vi "Detect Saccades (Messy w Graph).vi"(8 "error in (no error)":errorcluster, 9 "Config":T1={"N Samples"=10, "Thresh Acc Min"=2000.0, "Thresh Acc Mult"=1.3, "Biphasic Condition"=1.5} {"Biphasic Condition" format="%#_13g"; "Thresh Acc Min" format="%#_13g"}, 10 "Sample Rate (Hz)":dbl=500.0, 11 "Velocity Data":dbl[](array[numeric])=[4.667303200298225, 4.909677731146953, 5.2109745814792365, 5.55763581565099, 5.920839247626144, 6.2599375275868905, 6.53696746567776, 6.72865184750785, 6.832732456031344, 6.865145184809078, 6.858206597001612, 6.855560991647909, 6.9019024854844275, 7.042027036538185, 7.301808557734746, 7.67879884433365, 8.162701363544402, 8.739894904566324, 9.381804070066359, 10.060971955287894, 10.76783422583134, 11.502246410072347, 12.262929879380705, 13.045081013541676, 13.853884817610783, 14.695951720056332, 15.571765573591499, 16.488535497561312, 17.454938324359695, 18.484011737786314, 19.593891983853432, 20.806854336741793, 22.151712241900537, 23.654011428085493, 25.337827690951034, 27.230327185694577, 29.362424125147363, 31.75316688648706, 34.39263748770516, 37.23987577100237, 40.20998271205074, 43.18048939513237, 46.018360137909205, 48.61044269433803, 50.91951950237008, 53.06311795006367, 55.36174711261601, 58.34239623139827, 62.72019604358697, 69.31912993124544, 78.92734080431808, 92.11979839547627, 109.07789039502565, 129.463835379339, 152.35306948148417, 176.24888250277527, 199.24480922686814, 219.27781203835607, 234.41475989201246, 243.14123432233515, 244.61162292671878, 238.79626072654116, 226.47186493405752, 209.08996299834854, 188.54095925571488, 166.85076670397655, 145.88590014607087, 127.10744294855878, 111.41329184954873, 99.10408789193212, 89.94838177953986, 83.32435573521803, 78.40945230557072, 74.36256040478978, 70.48301661914127, 66.30206830018594, 61.60225100109197, 56.40307274892831, 50.896616982148316, 45.35594505323262, 40.04915633283459, 35.188143251090374, 30.904438051178893, 27.239307747637383, 24.160247711926996, 21.591099822449937, 19.444244062457226, 17.63526417873216, 16.092631691774315, 14.772784905414664, 13.652421403949939, 12.714696659266576, 11.949486890601628, 11.345398431951562, 10.88883280531385, 10.5770353190049, 10.405836535787293, 10.356779466571126, 10.406311733622601, 10.524935218461192, 10.678830860111066, 10.826005759205444, 10.907035432214682, 10.871451934497463, 10.694375519365607, 10.368230576729, 9.920494644655006, 9.421715176905362, 8.966350342238707, 8.642097141771771, 8.514860672075699, 8.617942426550648, 8.924287001994747, 9.353183534744435, 9.799968965203188, 10.152498912607701, 10.316635671318952, 10.249410666570771, 9.96446844667745, 9.529806688600937, 9.047812081889603, 8.616326801793129, 8.303617903780026, 8.136163116655617, 8.097459448535563, 8.12521569051474, 8.127278177630815, 8.019623108839935, 7.7527652198374994, 7.3178418750367875, 6.743220089832729, 6.091225621655573, 5.4388335182966125, 4.852885740463117, 4.374362223112637, 4.008624562640419, 3.726319072887119, 3.471108403172712, 3.176519977519715, 2.78491418737247, 2.2594461410939903, 1.59493884099372, 0.8181822934693148, -0.026619214287534554, -0.8813264042654012, -1.6754180023234415, -2.342793907914615, -2.8391064532580135, -3.1473600057829927, -3.2704346606176187, -3.2194026522732617, -3.015049071127091, -2.6913407449721714, -2.288963866373292, -1.8552012819132093, -1.4426441696461185, -1.10637493868746, -0.9037185529715961, -0.8855105498645095, -1.0878872191121767, -1.5222387174285608, -2.1642000966113475, -2.948745621863602, -3.774741677175757, -4.521225848850843, -5.0658752955379045, -5.311170309597713, -5.208438257945705, -4.772561349308287, -4.075895907311848, -3.2362701273178054, -2.4080793800097897, -1.7480331896475167, -1.3703588224237055, -1.3200274321352738, -1.5735992621749766, -2.042730927283582, -2.5851998693665657, -3.037924337271747, -3.256090588254791, -3.148166973862299, -2.6984451055504195, -1.9731790520825205, -1.1065567390523348, -0.2681141821144437, 0.37409311669090695, 0.6891756583069366, 0.6155860122500014, 0.17941599326467195, -0.5082906845765738, -1.2803499480545852, -1.9480888478483216, -2.3401497209829145, -2.3440992169137296, -1.9281270895302551, -1.1459474421566647, -0.12830962259723222, 0.9363738210892123, 1.8357991288182767, 2.384599745817786, 2.4666064308939344, 2.054156463248786, 1.220863305309523, 0.12811068784634827, -1.018595010969218, -2.001752664406064, -2.6304649399676983, -2.7869433851410292, -2.4535594735302872, -1.7140485905140306, -0.7334883840388606, 0.27392426391968705, 1.094585023452499, 1.5568403033256075, 1.5611234362432445, 1.0986668385472989, 0.24684742597984943, -0.8452725331409354, -1.9880582489864462, -2.9877533974319324, -3.6879053692364785, -4.00617610589776, -3.9395155261628396, -3.5545628002925387, -2.964302429928681, -2.3045670045288436, -1.7128444883759233, -1.294689818423599, -1.105155718562152, -1.1485119963907628, -1.3895741513688282, -1.7715422803726764, -2.2274763350570232, -2.6932733895783443, -3.113940417779075, -3.45287905028652, -3.70267849231551, -3.8744215557206916, -3.9856590761507915, -4.052808173290114, -4.09332504597233, -4.127471814491399, -4.167454556957223, -4.213014549974331, -4.258926261854726, -4.300292567500452, -4.332119774166569, -4.355168465827725, -4.374979301903575, -4.394294193594332, -4.415209965022706, -4.441144186890184, -4.467481232862541, -4.483248995233593, -4.4855721436010825, -4.4746031408485205, -4.450689654707525, -4.422434151675683, -4.403223628429705, -4.405917482243676, -4.4399518225329295, -4.512143144357493, -4.622080929076186, -4.757550150950738, -4.8958998491602115, -5.008497957121103, -5.0656431974498695, -5.039159628319716, -4.911773985777418, -4.678249782158317]) -> (0 "error out":errorcluster, 3 "Saccades":T2[](array[typedef]))   [LabVIEW 2016]
uses:
  Type Definitions/Saccade Analyser Saccade Data.ctl
  <vilib>/Analysis/NI_AALPro.lvlib
  <vilib>/Analysis/NI_AAL_SigProc.lvlib
  <vilib>/ptbypt/NI_PtbyPt.lvlib
panel:
  out "XY Graph":cluster{"Ramp (s)":dbl[], "dX/dt":dbl[]}[](graph)
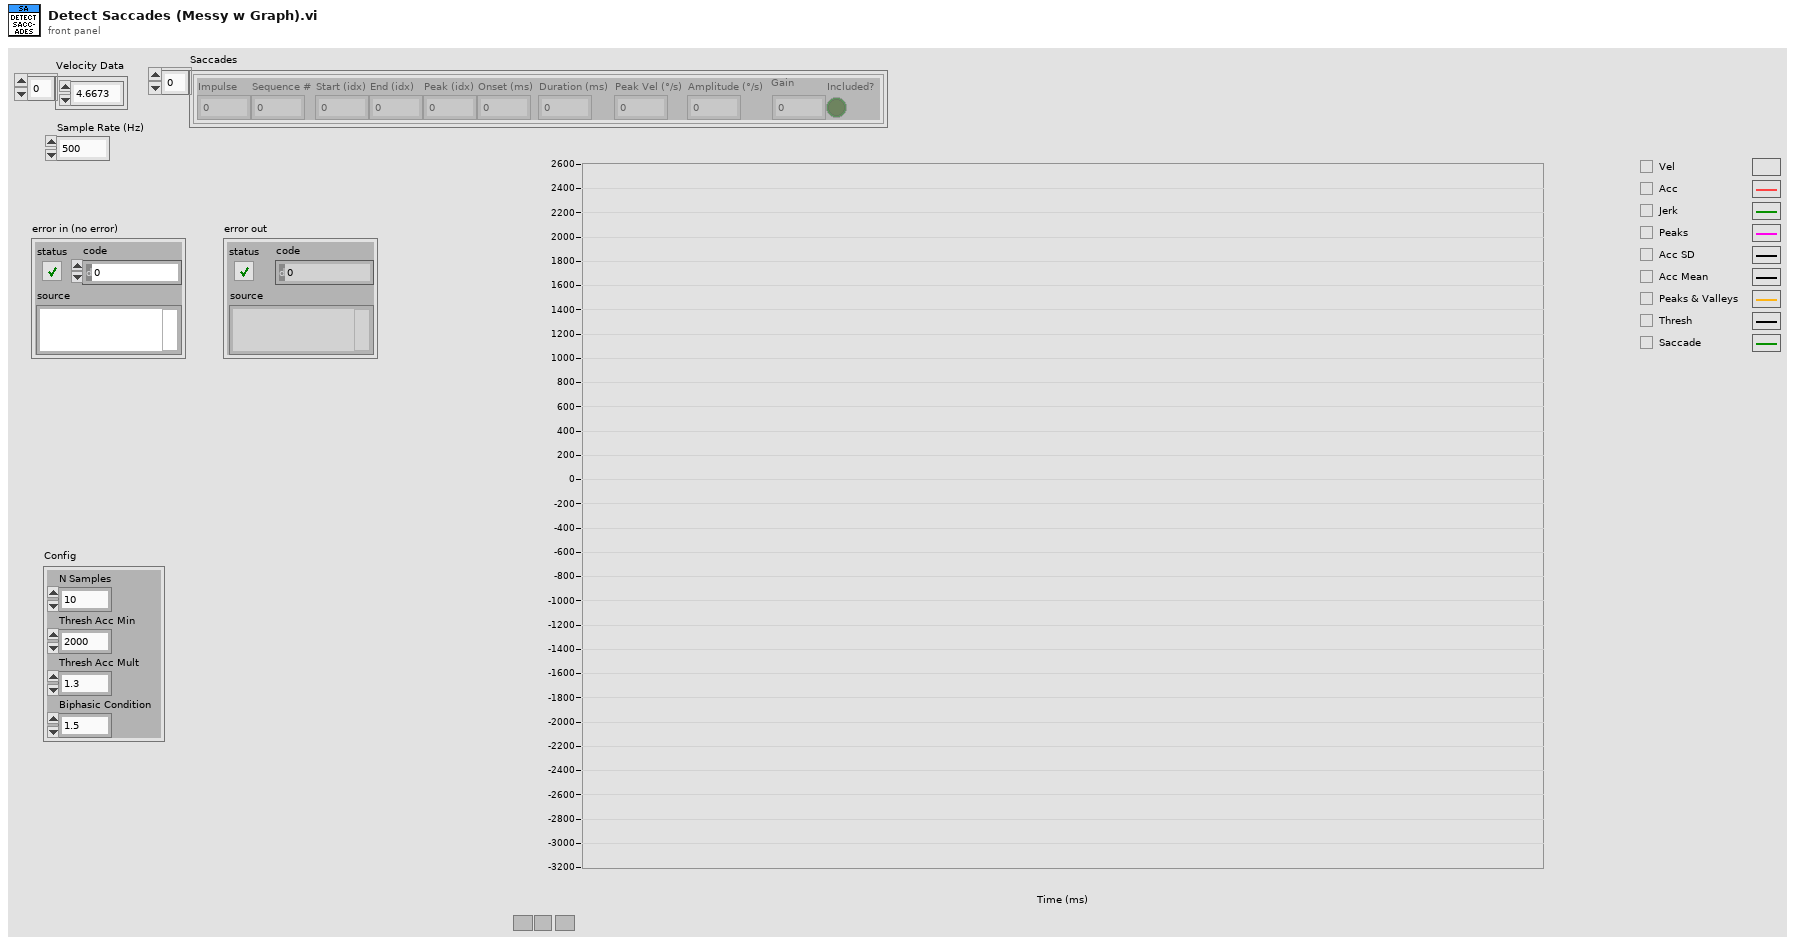
[diagram p1: front panel]
types:
  T1 = cluster{"N Samples":i32, "Thresh Acc Min":dbl, "Thresh Acc Mult":dbl, "Biphasic Condition":dbl}
  T2 = typedef "Saccade Analyser Saccade Data.ctl" = cluster{"Impulse":i32, "Sequence #":dbl, "Start (idx)":dbl, "End (idx)":dbl, "Peak (idx)":dbl, "Onset (ms)":dbl, "Duration (ms)":dbl, "Peak Vel (°/s)":dbl, "Amplitude (°/s)":dbl, "Gain":dbl, "Included?":bool}
  T3 = cluster{"Index":i32, "Peak?":bool, "Value":dbl}[]
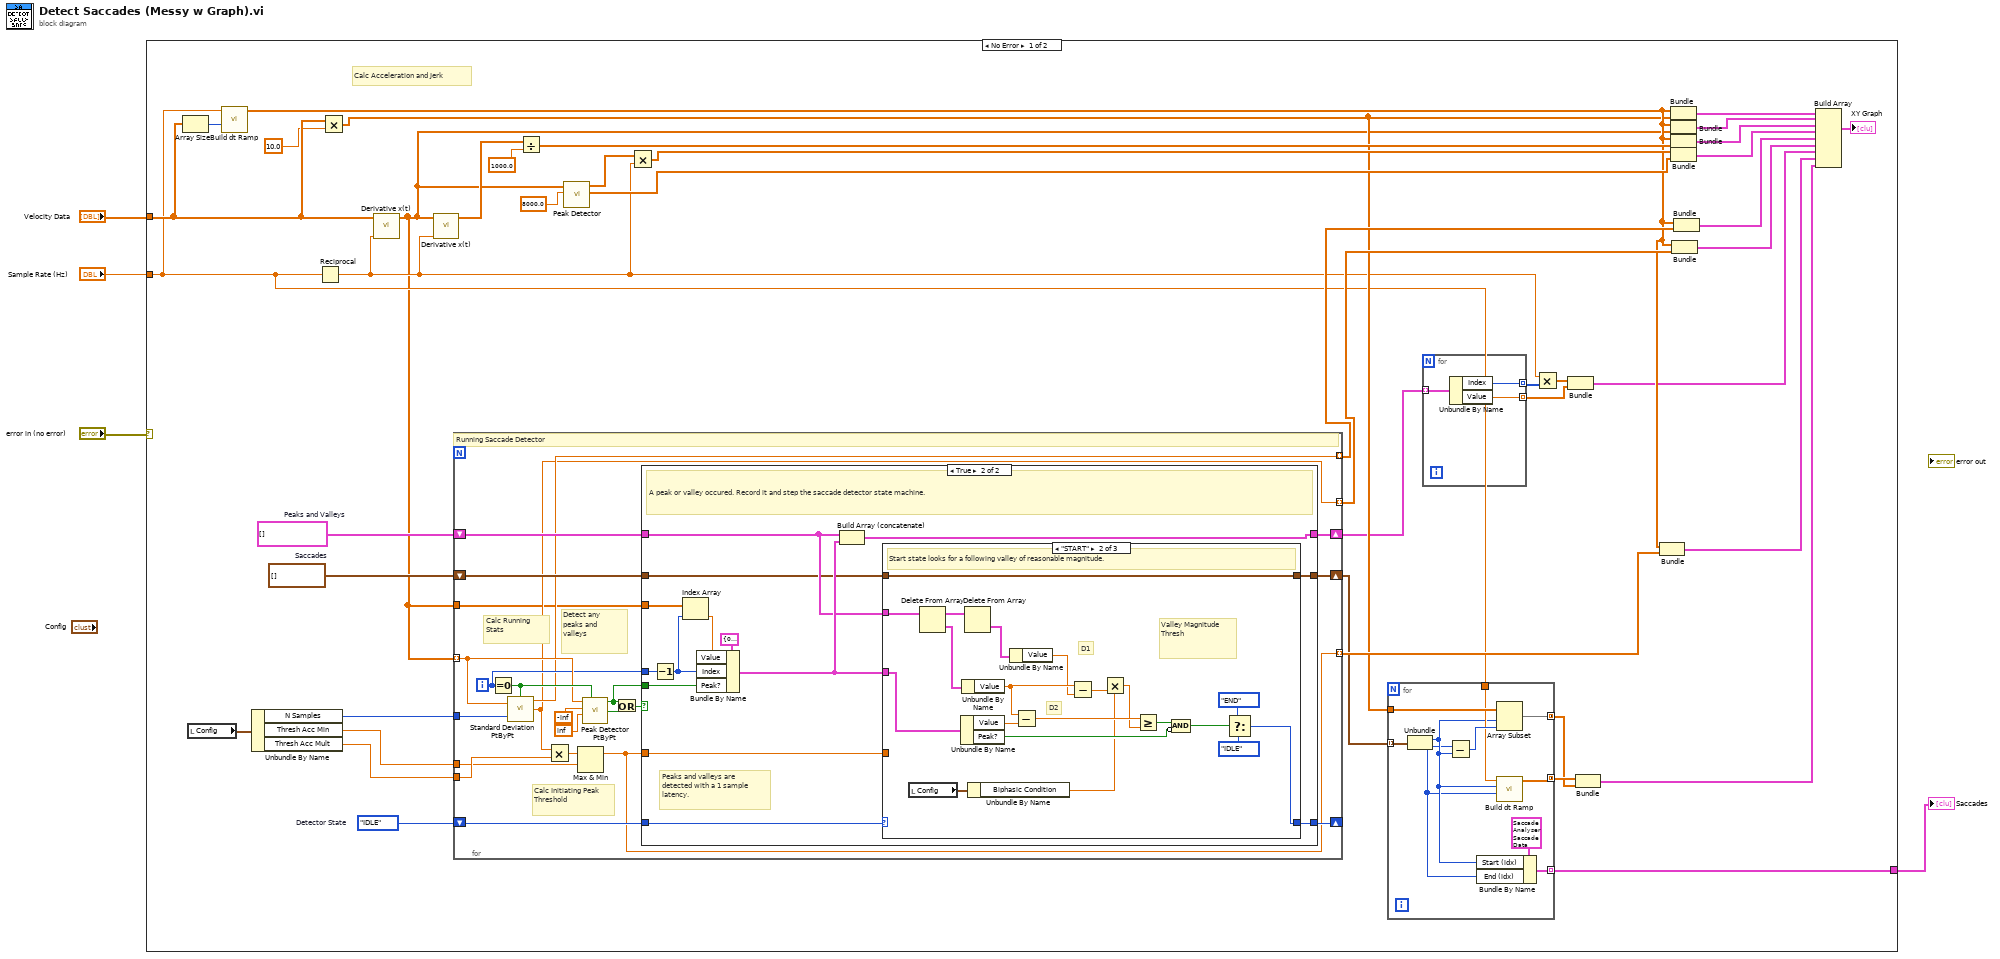
[diagram p0: block diagram]
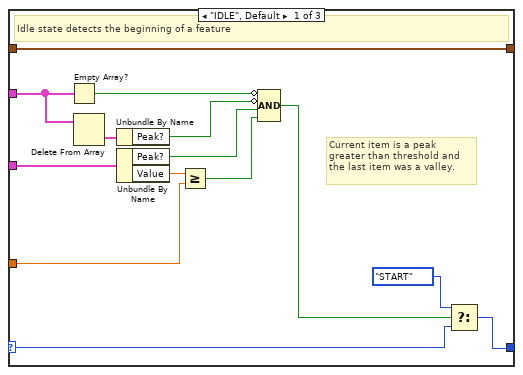
[diagram p3: hidden frame]
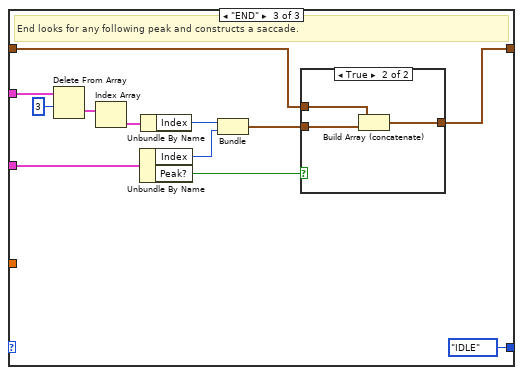
[diagram p4: hidden frame]
diagram:
  n1 = case shown="No Error" "error in (no error)" {
    tunnel: "Velocity Data" -> [w30 _]
    tunnel: "Sample Rate (Hz)" -> [w20 _]
    tunnel: [w9 _] -> w1
    frame No Error {
      w23 = cluster{"Start Index":i32, "End Index":i32}[] []  # Saccades
      w25 = enum16{"IDLE", "START", "END"}."IDLE"  # Detector State
      w24 = T3 []  # Peaks and Valleys
      # "Calc Acceleration and Jerk"
      n2 = Array Size(array=w30) -> (size(s)=w40:i32)
      n3 = local read "Config"() -> (w8:T1)
      n4 = call "Build dt Ramp.vi"("Stop idx"=w40, "Frequency (Hz)"=w20) -> ("Ramp (s)"=w28:dbl[])  [unwired: 8 in, 1 out]
      n5 = Unbundle By Name(w8) -> ("N Samples"=w7:i32, "Thresh Acc Min"=w6:dbl, "Thresh Acc Mult"=w5:dbl)
      n6 = Reciprocal(x=w20) -> (1/x=w14:dbl)
      n7 = Multiply(x=w30, y=10.0) -> (x*y=w21:dbl[])
      n8 = call <vilib>:"Derivative x(t).vi"("dt"=w14, "X"=w30) -> ("dX/dt"=w10:dbl[])  [unwired: 8 in, 1 out]
      n9 = call <vilib>:"Derivative x(t).vi"("dt"=w14, "X"=w10) -> ("dX/dt"=w43:dbl[])  [unwired: 8 in, 1 out]
      n10 = for {
        tunnel: w10 -> [w61] mode=indexing
        tunnel: w7 -> [w69]
        tunnel: w5 -> [w63]
        tunnel: w6 -> [w62]
        shift-right: [w65] -> _
        shift-left: w25 -> [w66]
        shift-right: [w59] -> w16
        shift-left: w24 -> [w60]
        shift-right: [w54] -> w22
        shift-left: w23 -> [w55]
        tunnel: [w53] -> w35 mode=indexing
        tunnel: [w52] -> w34 mode=indexing
        tunnel: [w51] -> w27 mode=indexing
        tunnel: w10 -> [w50]
        i -> [w57]
        # "Calc Initiating Peak Threshold"
        # "Detect any peaks and valleys"
        # "Calc Running Stats"
        # "Running Saccade Detector"
        n11 = Equal To 0?(x=w57) -> (x = 0?=w68:bool)
        n12 = call <vilib>:"Standard Deviation PtByPt.vi"("x"=w61, "sample length"=w69, "initialize"=w68) -> ("standard deviation"=w53:dbl, "mean"=w52:dbl)  [unwired: 1 out]
        n13 = Multiply(x=w52, y=w63) -> (x*y=w64:dbl)
        n14 = Max & Min(x=w64, y=w62) -> (max(x,y)=w51:dbl)  [unwired: 1 out]
        n15 = call <vilib>:"Peak Detector PtByPt.vi"("x"=w61, "threshold peak"=-inf, "threshold valley"=inf, "initialize"=w68) -> ("peak"=w56:bool, "valley"=w58:bool)  [unwired: 1 in, 1 out]
        n16 = Or(x=w56, y=w58) -> (x .or. y?=w67:bool)
        n17 = case shown="True" w67 {
          tunnel: w66 -> [w72 w86]
          tunnel: [w72 w78] -> w65
          tunnel: w51 -> [_ w83]
          tunnel: w60 -> [w71 w79]
          tunnel: [w71 w85] -> w59
          tunnel: w56 -> [_ w80]
          tunnel: w57 -> [_ w84]
          tunnel: w55 -> [w70 w77]
          tunnel: [w70 w76] -> w54
          tunnel: w50 -> [_ w75]
          frame False {
            # "A peak or valley did not occur. Do nothing."
          }
          frame True {
            # "Peaks and valleys are detected with a 1 sample latency."
            # "A peak or valley occured. Record it and step the saccade detector state machine."
            n18 = Decrement(x=w84) -> (x-1=w74:i32)
            n19 = Index Array(array=w75, index=w74) -> (element=w73:dbl)
            n20 = Bundle By Name(cluster=cluster{"Index":i32, "Peak?":bool, "Value":dbl} {"Index"=0, "Peak?"=FALSE, "Value"=0.0} ("Peak/Valley"), "Value"=w73, "Index"=w74, "Peak?"=w80) -> (w82:cluster{"Index":i32, "Peak?":bool, "Value":dbl})
            n21 = Build Array (concatenate)(w79, w82) -> (w85:T3)
            n22 = case shown="\"START\"" w86 {
              selector: w86 -> [w90 _ _]
              tunnel: w83 -> [w93 _ _]
              tunnel: w82 -> [w96 w116 w131]
              tunnel: w79 -> [w99 w120 w130]
              tunnel: [w88 w104 enum16{"IDLE", "START", "END"}."IDLE" ("Detector State")] -> w78
              tunnel: w77 -> [w87 w103 w126]
              tunnel: [w87 w103 w125] -> w76
              frame "IDLE", Default {
                # "Current item is a peak greater than threshold and the last item was a valley."
                # "Idle state detects the beginning of a feature"
                n23 = Empty Array?(array=w99) -> (empty?=w97:bool)
                n24 = Delete From Array(array=w99) -> (deleted portion=w100:cluster{"Index":i32, "Peak?":bool, "Value":dbl})  [unwired: 2 in, 1 out]
                n25 = Unbundle By Name(w100) -> ("Peak?"=w98:bool)
                n26 = Unbundle By Name(w96) -> ("Peak?"=w95:bool, "Value"=w94:dbl)
                n27 = Greater Or Equal?(x=w94, y=w93) -> (x >= y?=w92:bool)
                n28 = Compound Arithmetic op=AND(invert w97, invert w98, w95, w92) -> (w91:bool)
                n29 = Select(t=enum16{"IDLE", "START", "END"}."START" ("Detector State"), s=w91, f=w90) -> (s? t:f=w88:enum16{"IDLE", "START", "END"})
              }
              frame "START" {
                # "Valley Magnitude Thresh"
                # "D1"
                # "D2"
                # "Start state looks for a following valley of reasonable magnitude."
                n30 = local read "Config"() -> (w102:T1)
                n31 = Delete From Array(array=w120) -> (deleted portion=w118:cluster{"Index":i32, "Peak?":bool, "Value":dbl}, array with subset deleted=w119:T3)  [unwired: 2 in]
                n32 = Unbundle By Name(w116) -> ("Value"=w115:dbl, "Peak?"=w108:bool)
                n33 = Unbundle By Name(w118) -> ("Value"=w114:dbl)
                n34 = Delete From Array(array=w119) -> (deleted portion=w117:cluster{"Index":i32, "Peak?":bool, "Value":dbl})  [unwired: 2 in, 1 out]
                n35 = Unbundle By Name(w102) -> ("Biphasic Condition"=w101:dbl)
                n36 = Unbundle By Name(w117) -> ("Value"=w113:dbl)
                n37 = Subtract(x=w114, y=w115) -> (x-y=w112:dbl)
                n38 = Subtract(x=w114, y=w113) -> (x-y=w111:dbl)
                n39 = Multiply(x=w101, y=w111) -> (x*y=w110:dbl)
                n40 = Greater Or Equal?(x=w112, y=w110) -> (x >= y?=w109:bool)
                n41 = Compound Arithmetic op=AND(w109, invert w108) -> (w107:bool)
                n42 = Select(t=enum16{"IDLE", "START", "END"}."END" ("Detector State"), s=w107, f=enum16{"IDLE", "START", "END"}."IDLE" ("Detector State")) -> (s? t:f=w104:enum16{"IDLE", "START", "END"})
              }
              frame "END" {
                # "End looks for any following peak and constructs a saccade."
                n43 = Delete From Array(array=w130, length=3) -> (deleted portion=w128:T3)  [unwired: 1 in, 1 out]
                n44 = Index Array(array=w128) -> (element=w127:cluster{"Index":i32, "Peak?":bool, "Value":dbl})  [unwired: 1 in]
                n45 = Unbundle By Name(w131) -> ("Index"=w123:i32, "Peak?"=w121:bool)
                n46 = Unbundle By Name(w127) -> ("Index"=w124:i32)
                n47 = Bundle("Index"=w124, "Index"=w123) -> (w122:cluster{"Index":i32, "Index":i32})  [unwired: 1 in]
                n48 = case shown="True" w121 {
                  tunnel: w126 -> [w133 w136]
                  tunnel: [w133 w135] -> w125
                  tunnel: w122 -> [_ w134]
                  frame False {
                  }
                  frame True {
                    n49 = Build Array (concatenate)(w136, w134) -> (w135:cluster{"Index":i32, "Index":i32}[])
                  }
                }
              }
            }
          }
        }
      }
      n50 = Divide(x=w43, y=1000.0) -> (x/y=w41:dbl[])
      n51 = call <vilib>:"Peak Detector.vi"("threshold"=8000.0, "X"=w10) -> ("Amplitudes"=w31:dbl[], "Locations"=w37:dbl[])  [unwired: 5 in, 3 out]
      n52 = Multiply(x=w37, y=w14) -> (x*y=w36:dbl[])
      n53 = for {
        tunnel: w22 -> [w148] mode=indexing
        tunnel: w21 -> [w149]
        tunnel: w20 -> [w146]
        tunnel: [w145] -> w19 mode=concatenating
        tunnel: [w144] -> w18 mode=concatenating
        tunnel: [w140] -> w9 mode=indexing
        n54 = Unbundle(w148) -> ("Start Index"=w142:i32, "End Index"=w141:i32)
        n55 = Subtract(x=w141, y=w142) -> (x-y=w147:i32)
        n56 = Bundle By Name(cluster=T2 {"Impulse"=0, "Sequence #"=0.0, "Start (idx)"=0.0, "End (idx)"=0.0, "Peak (idx)"=0.0, "Onset (ms)"=0.0, "Duration (ms)"=0.0, "Peak Vel (°/s)"=0.0, "Amplitude (°/s)"=0.0, "Gain"=0.0, "Included?"=FALSE} ("Saccade"), "Start (idx)"=w142, "End (idx)"=w141) -> (w140:T2)
        n57 = Array Subset(array=w149, index=w142, length=w147) -> (w144:dbl[])
        n58 = call "Build dt Ramp.vi"("Stop idx"=w141, "Start idx (0)"=w142, "Frequency (Hz)"=w146) -> ("Ramp (s)"=w145:dbl[])  [unwired: 7 in, 1 out]
      }
      n59 = for {
        tunnel: w16 -> [w139] mode=indexing
        tunnel: [w138] -> w15 mode=indexing
        tunnel: [w137] -> w12 mode=indexing
        n60 = Unbundle By Name(w139) -> ("Index"=w138:i32, "Value"=w137:dbl)
      }
      n61 = Multiply(x=w14, y=w15) -> (x*y=w13:dbl[])
      n62 = Bundle(w13, w12) -> (w11:cluster{dbl[], dbl[]})  [unwired: 1 in]
      n63 = Bundle("Ramp (s)"=w19, w18) -> (w17:cluster{"Ramp (s)":dbl[], dbl[]})  [unwired: 1 in]
      n64 = Bundle("Ramp (s)"=w28, w27) -> (w26:cluster{"Ramp (s)":dbl[], dbl[]})  [unwired: 1 in]
      n65 = Bundle("Ramp (s)"=w28, w21) -> (w47:cluster{"Ramp (s)":dbl[], dbl[]})  [unwired: 1 in]
      n66 = Bundle("Ramp (s)"=w28, "dX/dt"=w10) -> (w46:cluster{"Ramp (s)":dbl[], "dX/dt":dbl[]})  [unwired: 1 in]
      n67 = Bundle("Ramp (s)"=w28, w41) -> (w45:cluster{"Ramp (s)":dbl[], dbl[]})  [unwired: 1 in]
      n68 = Bundle(w36, "Amplitudes"=w31) -> (w39:cluster{dbl[], "Amplitudes":dbl[]})  [unwired: 1 in]
      n69 = Bundle("Ramp (s)"=w28, w34) -> (w32:cluster{"Ramp (s)":dbl[], dbl[]})  [unwired: 1 in]
      n70 = Bundle("Ramp (s)"=w28, w35) -> (w33:cluster{"Ramp (s)":dbl[], dbl[]})  [unwired: 1 in]
      n71 = Build Array(w47, w46, w45, w39, w33, w32, w11, w26, w17) -> (→"XY Graph":cluster{"Ramp (s)":dbl[], "Amplitudes":dbl[]}[])
    }
    frame Error {
    }
  }
  "Saccades" <- w1
